vi "MakeSegmentThinClientExample.vi"() -> ()   [LabVIEW 2015]
uses:
  <vilib>/MDSplus_LV2015/Library/MDSplus.lvlib
panel:
  in  "Path":string
  in  "Shot":i32
  in  "Tree":string
  in  "IP:port":string
  out "Overall Waveform":sgl[](graph)
  out "Waveform Graph":dynamicdata(graph)
  in  "stop":bool
  in  "phase":dbl
  in  "amplitude":dbl=5.0
  in  "frequency":dbl=1.1
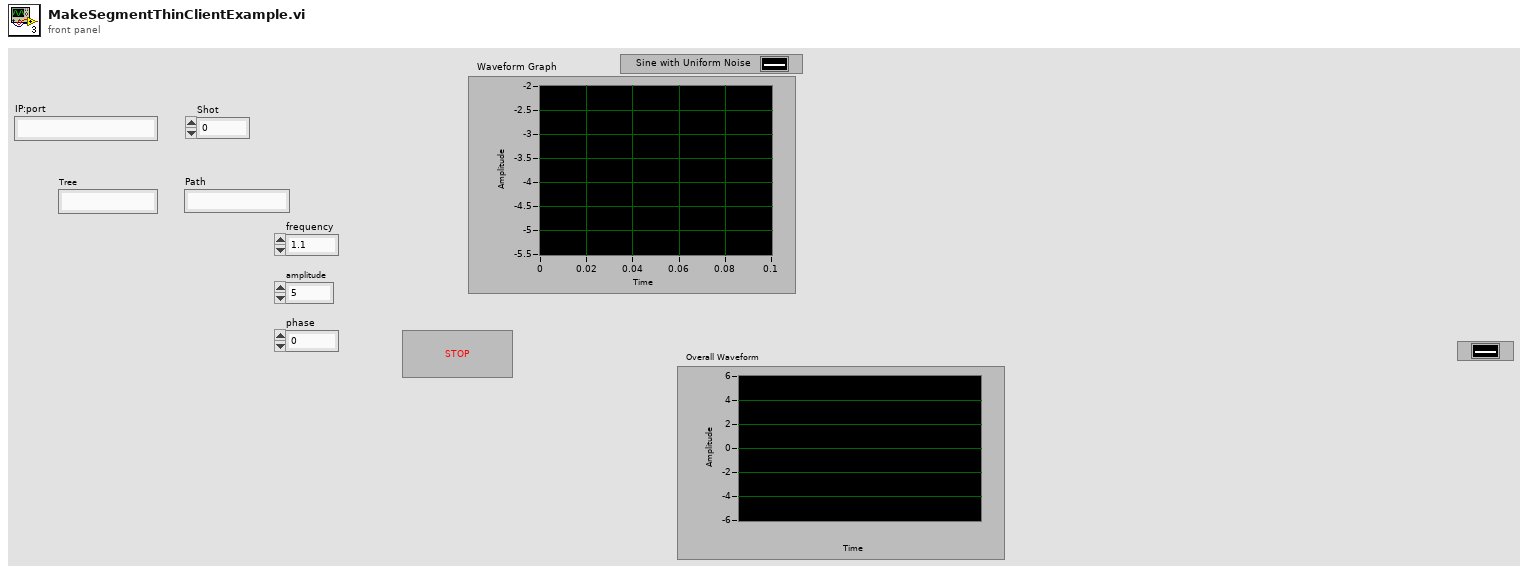
[diagram p1: front panel]
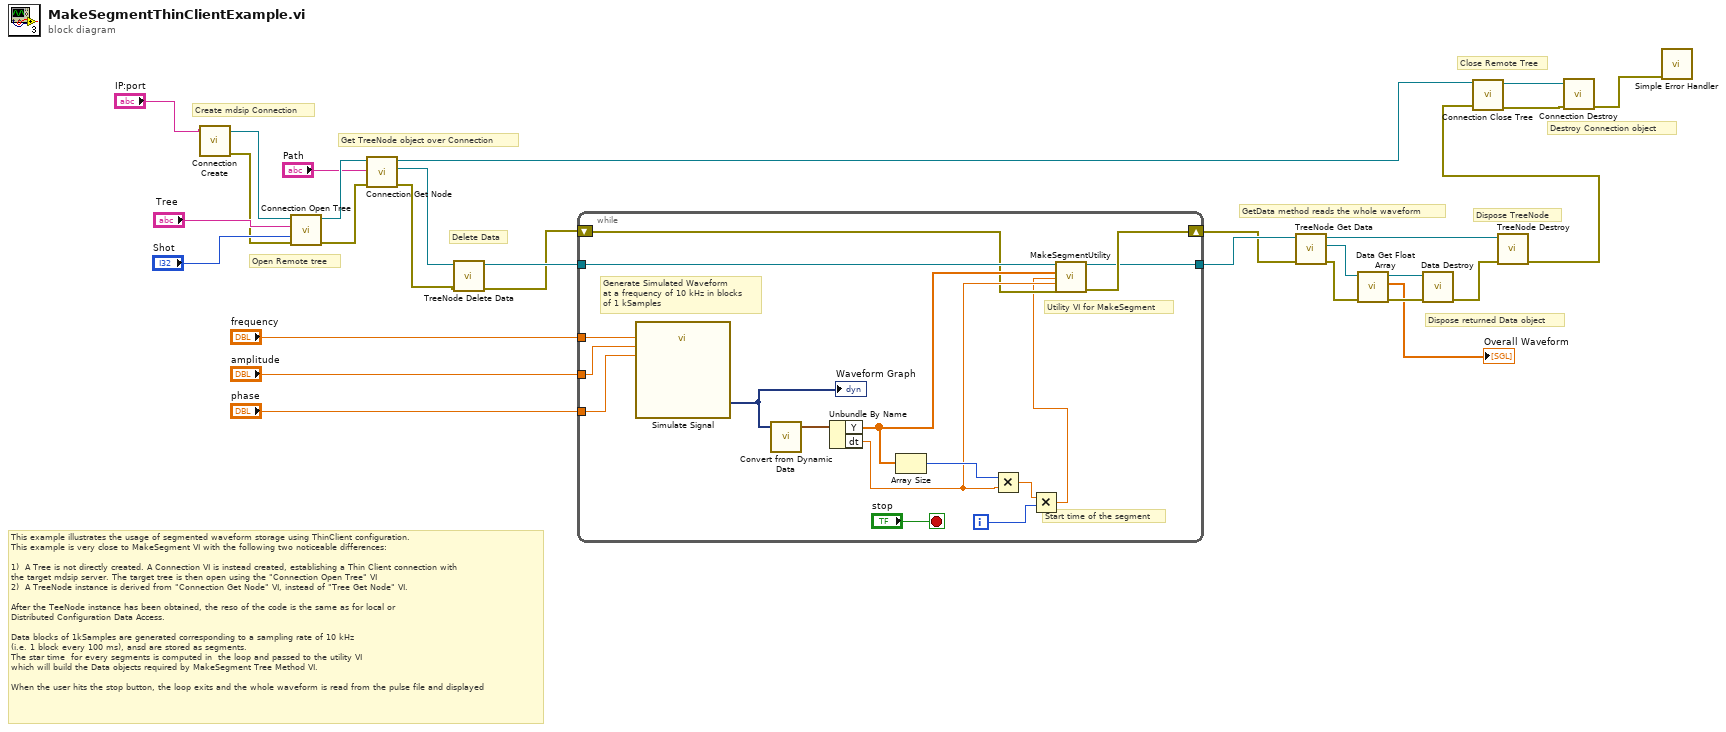
[diagram p0: block diagram]
diagram:
  # "Destroy Connection object"
  # "Close Remote Tree"
  # "Get TreeNode object over Connection"
  # "Open Remote tree"
  # "Create mdsip Connection"
  # "Dispose TreeNode"
  # "GetData method reads the whole waveform"
  # "Dispose returned Data object"
  # "This example illustrates the usage of segmented waveform storage using ThinClient configuration. \nThis example is very close to MakeSegment VI with the following two noticeable differences:\n\n1)  A Tree is not directly created. A Connection VI is instead created, establishing a Thin Client connection with \nthe target mdsip server. The target tree is then open using the \"Connection Open Tree\" VI\n2)  A TreeNode instance is derived from \"Connection Get Node\" VI, instead of \"Tree Get Node\" VI.\n   \nAfter the TeeNode instance has been obtained, the reso of the code is the same as for local or \nDistributed Configuration Data Access.\n\nData blocks of 1kSamples are generated corresponding to a sampling rate of 10 kHz\n(i.e. 1 block every 100 ms), ansd are stored as segments. \nThe star time  for every segments is computed in  the loop and passed to the utility VI\nwhich will build the Data objects required by MakeSegment Tree Method VI. \n\nWhen the user hits the stop button, the loop exits and the whole waveform is read from the pulse file and displayed"
  # "Delete Data"
  n1 = call <vilib>:"Connection Create.vi"("Ip : port"="IP:port") -> ("error out"=w11:errorcluster, "Connection DVR out"=w14:refnum<data-value>)  [unwired: 9 in]
  n2 = call <vilib>:"Connection Open Tree.vi"("error in (no error)"=w11, "Shot"="Shot", "Tree"="Tree", "Connection DVR in"=w14) -> ("error out"=w8:errorcluster, "Connection DVR out"=w10:refnum<data-value>)  [unwired: 6 in]
  n3 = call <vilib>:"Connection Get Node.vi"("error in (no error)"=w8, "Path in"="Path", "Connection DVR in"=w10) -> ("error out"=w6:errorcluster, "Node out"=w7:refnum<data-value>, "Connection DVR out"=w2:refnum<data-value>)  [unwired: 6 in]
  n4 = call <vilib>:"TreeNode Delete Data.vi"("error in (no error)"=w6, "TreeNode DVR in"=w7) -> ("error out"=w16:errorcluster, "TreeNode DVR out"=w17:refnum<data-value>)  [unwired: 8 in]
  n5 = while {
    tunnel: "frequency" -> [w44]
    tunnel: "amplitude" -> [w43]
    tunnel: "phase" -> [w42]
    shift-right: [w32] -> w18
    shift-left: w16 -> [w33]
    tunnel: w17 -> [w40]
    tunnel: [w31] -> w19
    i -> [w35]
    stop <- "stop" stop-if-true
    # "Utility VI for MakeSegment"
    # "Generate Simulated Waveform\nat a frequency of 10 kHz in blocks\nof 1 kSamples"
    # "Start time of the segment"
    n6 = call "Simulate Signal"("Frequency"=w44, "Amplitude"=w43, "Phase"=w42) -> ("Sine with Uniform Noise"=w41:dynamicdata)  [unwired: 11 in, 1 out]
    "Waveform Graph" <- w41
    n7 = call "Convert from Dynamic Data"("Dynamic Data Type"=w41) -> ("Waveform"=w39:waveform(dbl))  [unwired: 3 in]
    n8 = Unbundle By Name(w39) -> ("Y"=w38:dbl[], "dt"=w34:dbl)
    n9 = Array Size(array=w38) -> (size(s)=w37:i32)
    n10 = Multiply(x=w37, y=w34) -> (x*y=w36:dbl)
    n11 = Multiply(x=w36, y=w35) -> (x*y=w30:dbl)
    n12 = call <vilib>:"MakeSegmentUtility.vi"("TreeNode DVR in"=w40, "DBL Array"=w38, "Start time"=w30, "dt"=w34, "error in (no error)"=w33) -> ("TreeNode DVRout"=w31:refnum<data-value>, "error out"=w32:errorcluster)  [unwired: 9 in]
  }
  n13 = call <vilib>:"TreeNode Get Data.vi"("error in (no error)"=w18, "TreeNode DVR in"=w19) -> ("error out"=w24:errorcluster, "Data out"=w25:refnum<data-value>, "TreeNode DVR out"=w26:refnum<data-value>)  [unwired: 7 in]
  n14 = call <vilib>:"Data Get Float Array.vi"("error in (no error)"=w24, "Data DVR in"=w25) -> ("error out"=w23:errorcluster, "SGL array out"=→"Overall Waveform":sgl[], "Data DVR out"=w22:refnum<data-value>)  [unwired: 6 in, 1 out]
  n15 = call <vilib>:"Data Destroy.vi"("error in (no error)"=w23, "Data DVR in"=w22) -> ("error out"=w21:errorcluster)  [unwired: 9 in]
  n16 = call <vilib>:"TreeNode Destroy.vi"("error in (no error)"=w21, "TreeNode DVR in"=w26) -> ("error out"=w1:errorcluster)  [unwired: 9 in]
  n17 = call <vilib>:"Connection Close Tree.vi"("error in (no error)"=w1, "Connection DVR in"=w2) -> ("error out"=w4:errorcluster, "Connection DVR out"=w5:refnum<data-value>)  [unwired: 8 in]
  n18 = call <vilib>:"Connection Destroy.vi"("error in (no error)"=w4, "Connection DVR in"=w5) -> ("error out"=w3:errorcluster)  [unwired: 9 in]
  n19 = call <vilib>:"Simple Error Handler.vi"("error in (no error)"=w3) -> ()  [unwired: 4 in, 5 out]
